vi "Image_Summation.vi"() -> ()   [LabVIEW 2018]
uses:
  <vilib>/vision/NI_Vision_Development_Module.lvlib
panel:
  out "Image Pixels (U32) 2":u32[][](array[numeric])
  out "Image Pixels (U32)":u32[][](array[numeric])
  out "x+y":u32[][](array[numeric])
  in  "Image Name 2":string="untitled"
  out "error out":errorcluster
  out "Numeric 2":i32
  in  "name or relative path":i32
  in  "Numeric":i32
  in  "base path":path
  in  "Output":path
  in  "Image Name":string="untitled"
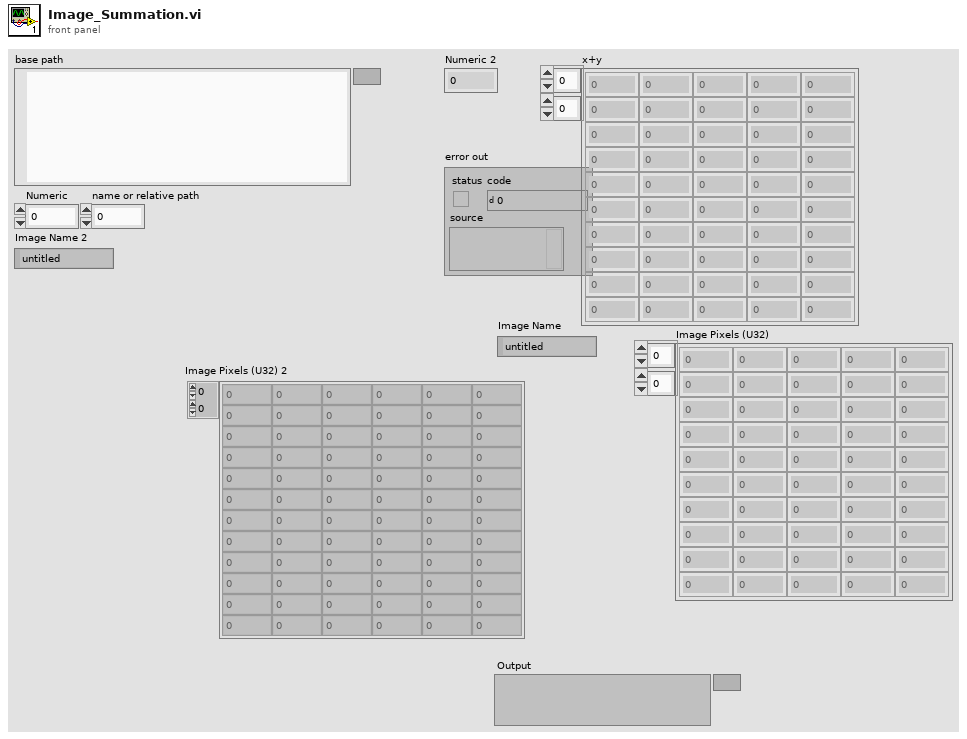
[diagram p1: front panel]
types:
  T1 = typedef "Image Type" = u32
  T2 = typedef "IMAQ Image.ctl" = refnum<image>
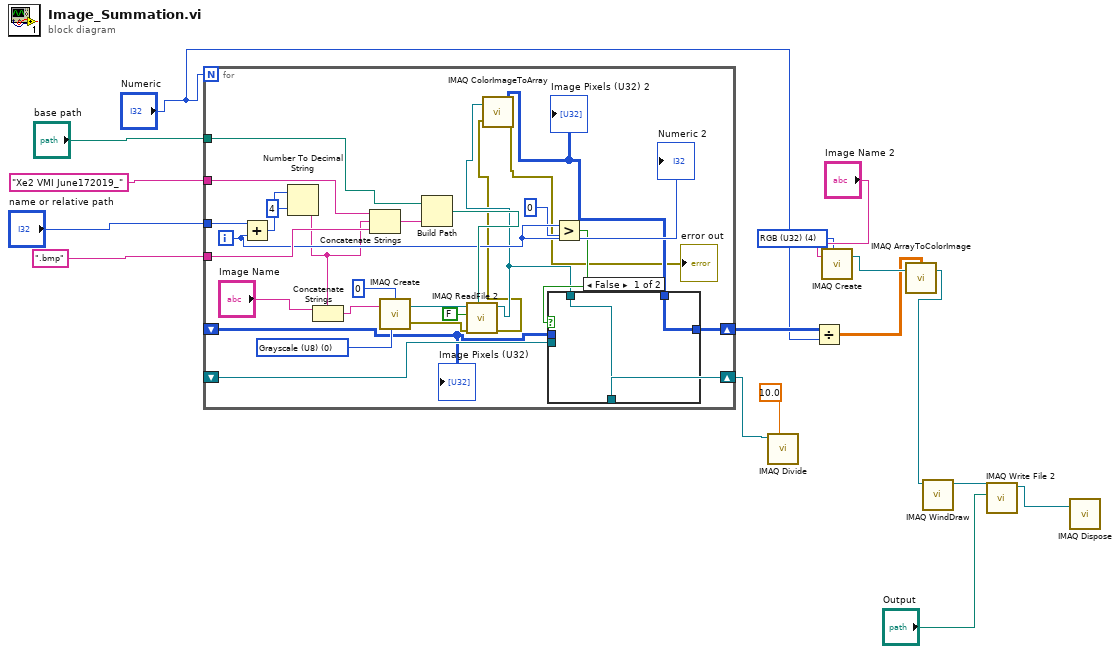
[diagram p0: block diagram]
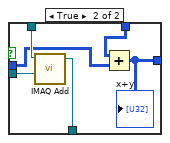
[diagram p2: hidden frame]
diagram:
  w4 = T1 4 items=["Grayscale (U8)", "Grayscale (I16)", "Grayscale (SGL)", "Complex (CSG)", "RGB (U32)", "HSL (U32)", "RGB (U64)", "Grayscale (U16)"] ("Image Type")
  n1 = for {
    N: "Numeric" -> [_]
    tunnel: "base path" -> [w40]
    tunnel: ".bmp" ("name or relative path") -> [w39]
    tunnel: "Xe2 VMI June172019_" ("string") -> [w37]
    tunnel: "name or relative path" -> [w35]
    shift-right: [w32] -> w9
    shift-left: _ -> [w31]
    shift-right: [w23] -> w8
    shift-left: _ -> [w22]
    i -> [w30]
    w42 = T1 0 items=["Grayscale (U8)", "Grayscale (I16)", "Grayscale (SGL)", "Complex (CSG)", "RGB (U32)", "HSL (U32)", "RGB (U64)", "Grayscale (U16)"] ("Image Type")
    n2 = Add(x=w35, y=w30) -> (x+y=w34:i32)
    n3 = Number To Decimal String(number=w34, width (-)=i16 4) -> (decimal integer string=w27:string)
    n4 = Concatenate Strings("Image Name", w27) -> (w25:string)
    n5 = Concatenate Strings(w37, w27, w39) -> (w38:string)
    n6 = call "IMAQ Create"("Border Size"=0, "Image Name"=w25, "Image Type"=w42) -> ("New Image"=w24:T2, "error out"=w41:errorcluster)  [unwired: 2 in]
    n7 = Build Path(base path=w40, name or relative path=w38) -> (appended path=w36:path)
    n8 = call "IMAQ ReadFile 2"("File Path"=w36, "error in (no error)"=w41, "Load Color Palette? (No)"=FALSE, "Image"=w24) -> ("error out"=w18:errorcluster, "Image Out"=w21:T2)  [unwired: 3 in, 3 out]
    n9 = call "IMAQ ColorImageToArray"("Image"=w21, "error in (no error)"=w18) -> ("Image Pixels (U32)"=w20:u32[][], "error out"=→"error out":errorcluster)  [unwired: 2 in, 1 out]
    "Image Pixels (U32) 2" <- w20
    n10 = Greater?(x=w30, y=0) -> (0:w28:bool)
    n11 = case shown="False" w28 {
      tunnel: [w45 w51] -> w32
      tunnel: w31 -> [_ w50]
      tunnel: w21 -> [w45 w49]
      tunnel: w20 -> [w44 w48]
      tunnel: [w44 w47] -> w23
      tunnel: w22 -> [_ w46]
      frame False {
      }
      frame True {
        n12 = call "IMAQ Add"("Image Src A"=w49, "Image Src B"=w50) -> ("Image Dst Out"=w51:T2)  [unwired: 5 in, 1 out]
        n13 = Add(x=w48, y=w46) -> (x+y=w47:u32[][])
        "x+y" <- w47
      }
    }
    "Numeric 2" <- w30
    "Image Pixels (U32)" <- w22
  }
  n14 = call "IMAQ Divide"("Image Src A"=w9, "Constant"=10.0) -> ()  [unwired: 5 in, 2 out]
  n15 = Divide(x=w8, y="Numeric") -> (x/y=w1:dbl[][])
  n16 = call "IMAQ Create"("Image Name"="Image Name 2", "Image Type"=w4) -> ("New Image"=w3:T2)  [unwired: 3 in, 1 out]
  n17 = call "IMAQ ArrayToColorImage"("Image Pixels (U32)"=w1, "Image"=w3) -> ("Image Out"=w2:T2)  [unwired: 3 in, 1 out]
  n18 = call "IMAQ WindDraw"("Image"=w2) -> ("Image Out (duplicate)"=w15:T2)  [unwired: 9 in, 1 out]
  n19 = call-poly "IMAQ Write File 2"("File Path"="Output", "Image"=w15) -> ("Image Out (duplicate)"=w14:T2)  [unwired: 8 in, 1 out]
  n20 = call "IMAQ Dispose"("Image"=w14) -> ()  [unwired: 5 in, 1 out]
